vi "AT Is Implemented A.vi"(8 "error in (no error)":errorcluster, 10 "Feature":string, 11 "Handle":i32) -> (0 "error out":errorcluster, 2 "Implemented":bool, 3 "Status":i32)   [LabVIEW 2009]
doc: "Is Implemented\n\nOutput:\n I32 Status\n Bool Implemented\n\nInput:\n I32 Handle\n String Feature\n\nThis function can be used to determine whether the camera has implemented the feature specified by the\nFeature parameter. On return the Implemented parameter will contain the value FALSE or TRUE. In the case that the feature is implemented the value of Implemented will be TRUE, otherwise it will be\nFALSE."
uses:
  atcoreA.dll
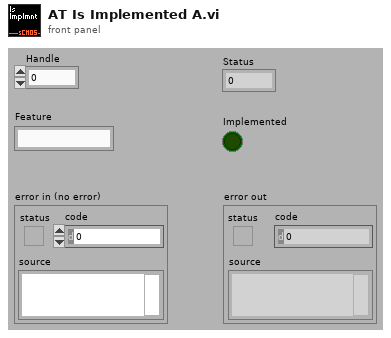
[diagram p1: front panel]
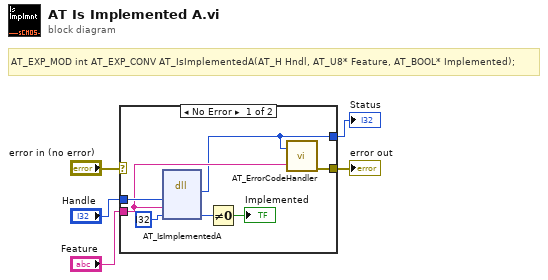
[diagram p0: block diagram]
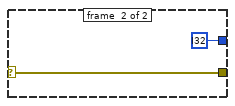
[diagram p2: hidden frame]
diagram:
  # "AT_EXP_MOD int AT_EXP_CONV AT_IsImplementedA(AT_H Hndl, AT_U8* Feature, AT_BOOL* Implemented);"
  n1 = case shown="No Error" "error in (no error)" {
    selector: "error in (no error)" -> [_ w14]
    tunnel: [w6 i32 ?] -> w5
    tunnel: "Handle" -> [w12 _]
    tunnel: "Feature" -> [w7 _]
    tunnel: [w8 w14] -> w2
    frame #0 {
      n2 = dll-call lib="atcoreA.dll" fn="AT_IsImplementedA"("Handle"=w12, "Feature"=w7, "Implemented"=i32 ?) -> ("Status"=w6:i32, "Implemented"=w9:i32)  [unwired: 5 in, 2 out]
      n3 = Not Equal To 0?(x=w9) -> (x != 0?=→"Implemented":bool)
      n4 = call "AT_ErrorCodeHandler.vi"("Error"=w6, "Feature Name"=w7) -> ("error out"=w8:errorcluster)  [unwired: 5 in]
    }
    frame #1 {
    }
  }
  "Status" <- w5
  "error out" <- w2
